vi "DIO Test.vi"() -> ()   [LabVIEW 2017]
panel:
  out "appended array":u32[](array[numeric])
  in  "Boolean array 2":bool[](array[boolean])
  in  "stop":bool
  out "Boolean array":bool[](array[boolean])
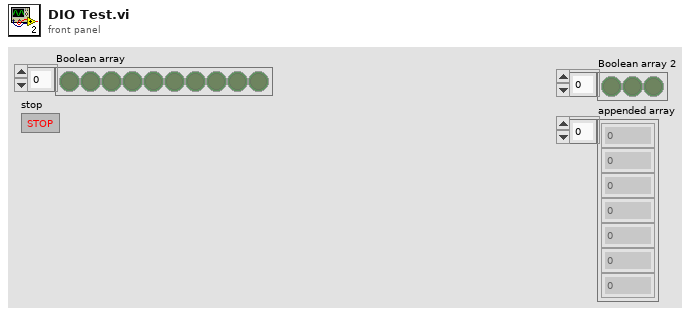
[diagram p1: front panel]
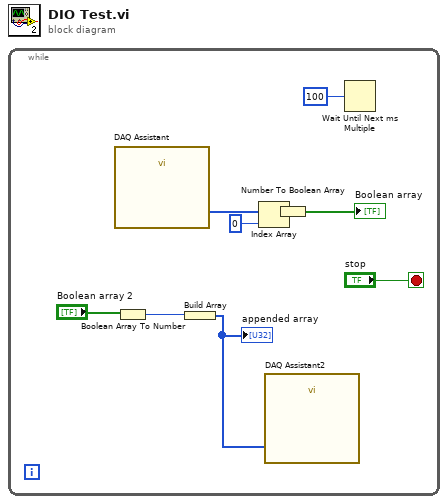
[diagram p0: block diagram]
diagram:
  n1 = while {
    stop <- "stop" stop-if-true
    n2 = call "DAQ Assistant"() -> ("data"=w9:u32[])  [unwired: 17 in, 2 out]
    n3 = Boolean Array To Number(Boolean array="Boolean array 2") -> (number=w2:u32)
    n4 = Build Array(w2) -> (w1:u32[])
    "appended array" <- w1
    n5 = Index Array(array=w9, index=0) -> (element=w7:u32)
    n6 = call "DAQ Assistant2"("data"=w1) -> ()  [unwired: 17 in, 2 out]
    n7 = Number To Boolean Array(number=w7) -> (Boolean array=→"Boolean array":bool[])
    n8 = Wait Until Next ms Multiple(millisecond multiple=u32 100) -> ()  [unwired: 1 out]
  }
